vi "Pattern Generator Pt by Pt_5734.vi"(7 "sampling info":cluster{"Fs":dbl, "#s":dbl}={"Fs"=250000000.0, "#s"=1000.0} {"Fs" format="%#_p"}, 9 "Marker Position":u32, 10 "signal type":T1(ring), 11 "Frequency":dbl=5000000.0 format="%0.2p") -> (1 "Wfm Counter":u32, 2 "Marker":bool, 3 "Data":i16(graph), 4 "Wfm":dbl[](array[numeric]))   [LabVIEW 2012]
uses:
  <vilib>/measure/NI_MABase.lvlib
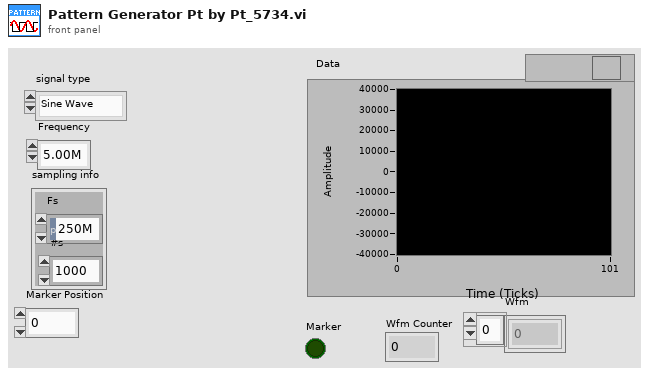
[diagram p1: front panel]
types:
  T1 = enum16{"Sine Wave", "Triangle Wave", "Square Wave", "Sawtooth Wave"}
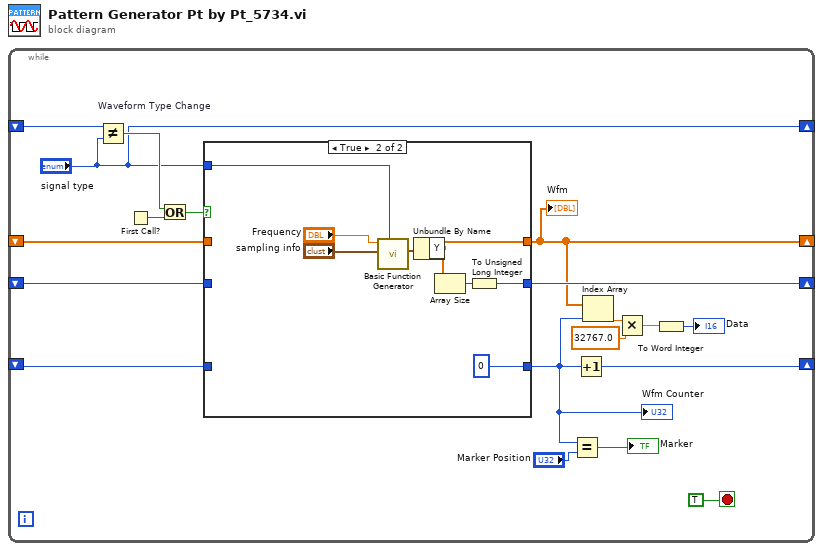
[diagram p0: block diagram]
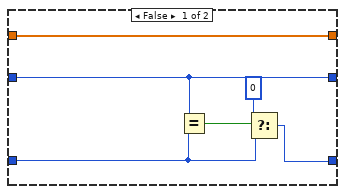
[diagram p2: hidden frame]
diagram:
  n1 = while {
    shift-right: [w6] -> _
    shift-left: _ -> [w15]
    shift-right: [w10] -> _
    shift-left: _ -> [w13]
    shift-right: [w12] -> _
    shift-left: _ -> [w11]
    shift-right: ["signal type"] -> _
    shift-left: _ -> [w5]
    stop <- TRUE ("stop") stop-if-true
    n2 = Not Equal? "Waveform Type Change"(x=w5, y="signal type") -> (x != y?=w3:bool)
    n3 = First Call?() -> (First Call?: T/F=w4:bool)
    n4 = Or(x=w3, y=w4) -> (x .or. y?=w2:bool)
    n5 = case shown="True" w2 {
      tunnel: [w25 w30] -> w6
      tunnel: w15 -> [w25 _]
      tunnel: w13 -> [w23 _]
      tunnel: [w21 w27] -> w12
      tunnel: w11 -> [w21 _]
      tunnel: [w22 u32 0] -> w7
      tunnel: "signal type" -> [_ w26]
      frame False {
        n6 = Equal?(x=w21, y=w23) -> (x = y?=w24:bool)
        n7 = Select(t=u32 0, s=w24, f=w23) -> (s? t:f=w22:u32)
      }
      frame True {
        n8 = call <vilib>:"Basic Function Generator.vi"("sampling info"="sampling info", "signal type"=w26, "frequency"="Frequency") -> ("signal out"=w33:waveform(dbl))  [unwired: 6 in, 2 out]
        n9 = Unbundle By Name(w33) -> ("Y"=w30:dbl[])
        n10 = Array Size(array=w30) -> (size(s)=w29:i32)
        n11 = To Unsigned Long Integer(number=w29) -> (unsigned 32bit integer=w27:u32)
      }
    }
    "Wfm Counter" <- w7
    "Wfm" <- w6
    n12 = Equal?(x=w7, y="Marker Position") -> (x = y?=→"Marker":bool)
    n13 = Increment(x=w7) -> (x+1=w10:u32)
    n14 = Index Array(array=w6, index=w7) -> (element=w14:dbl)
    n15 = Multiply(x=w14, y=32767.0) -> (x*y=w17:dbl)
    n16 = To Word Integer(number=w17) -> (16bit integer=→"Data":i16)
  }
